vi "Read ARTIQ Master Repo Path.vi"(8 "error in (no error)":errorcluster, 11 "Kasli in":refnum<class "Kasli.lvclass">) -> (0 "error out":errorcluster, 2 "ARTIQ Master Repo Path":string, 3 "Kasli out":refnum<class "Kasli.lvclass">)   [LabVIEW 2020, in "Kasli Wrapper 2.0.lvlib" / "Kasli.lvclass"]
uses:
  Kasli.lvclass
  Kasli.lvclass/Kasli.ctl
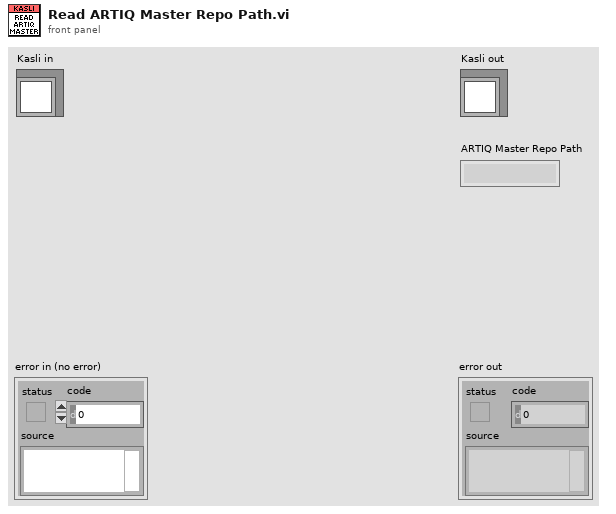
[diagram p1: front panel]
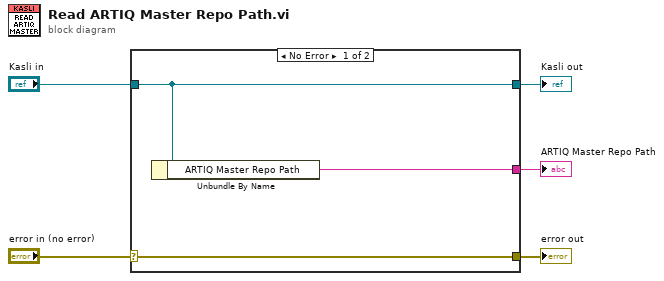
[diagram p0: block diagram]
diagram:
  n1 = case shown="No Error" "error in (no error)" {
    selector: "error in (no error)" -> [w8 w9]
    tunnel: [w8 w9] -> w4
    tunnel: [w7 w10] -> w2
    tunnel: "Kasli in" -> [w7 w10]
    tunnel: [w6 _] -> w1
    frame No Error {
      n2 = Unbundle By Name(w7) -> ("ARTIQ Master Repo Path"=w6:string)
    }
    frame Error {
    }
  }
  "error out" <- w4
  "Kasli out" <- w2
  "ARTIQ Master Repo Path" <- w1
